vi "Robot Global Data.vi"() -> ()   [LabVIEW 2019]
doc: "This global VI can contain as many global variables as you need. Place a control on the panel, give it a good name. To read or write to it from a VI, drag the icon to the diagram of that VI. You can also drag from the project. Click on the node to change which global you access. You shouldn't have multiple locations writing to a global or it will cause a race-condition."
uses:
  <vilib>/Rock Robotics/WPI/Camera/WPI_CameraImageSize.ctl
  <vilib>/Rock Robotics/WPI/DriverStation/WPI_DriverStationRobotMode2.ctl
panel:
  out "stall":bool
  out "tvert":dbl
  out "Intake C":bool
  in  "Shooter Lower":dbl
  in  "Shooter Top":dbl
  out "Beginning Yaw":dbl
  in  "Max Drive Power":dbl=0.9
  in  "Max Turn Power":dbl=0.55
  in  "log text":string
  out "Status":dbl
  in  "VISA Arduino name":refnum<visa-resource-name>
  out "Tape Height":dbl
  out "Tape X":dbl
  out "Camera Light":bool
  out "Heading":dbl
  out "Robot Y":dbl
  out "Robot X":dbl
  out "valid?":dbl
  out "targetArea":dbl
  out "yOffset":dbl
  out "xOffset":dbl
  in  "Robot Mode":T1
  in  "image size":T2=enum."320x240"
  in  "Enable Vision":bool
  # "Limelight"
  # "Pixy"
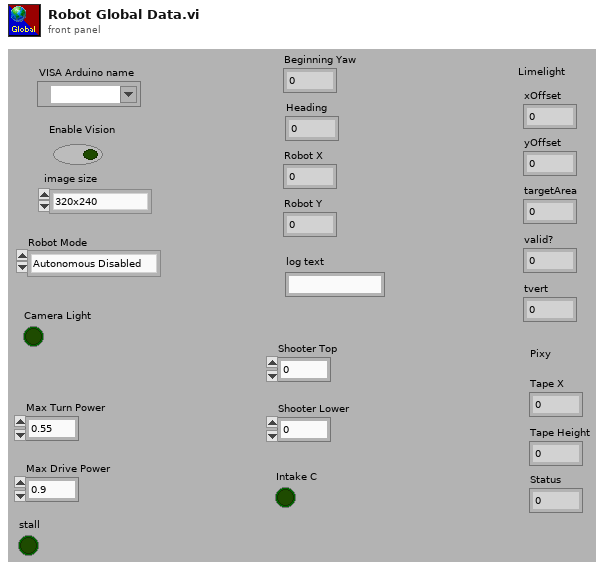
[diagram p1: front panel]
types:
  T1 = typedef "WPI_DriverStationRobotMode2.ctl" = enum16{"Autonomous Disabled", "Autonomous Enabled", "Teleop Disabled", "Teleop Enabled", "Disconnected", "Finish", "Test Disabled", "Test Enabled", "Emergency Stopped"}
  T2 = typedef "WPI_CameraImageSize.ctl" = enum16{"640x480", "320x240", "160x120", "Custom"}
diagram:
